vi "feature select.vi"(9 "Feature Selection":T1) -> (3 "VI Refnum":refnum<vi>)   [LabVIEW 2016, in "main.lvlib"]
doc: "Selects which reference is used"
uses:
  main.lvlib
  upper subpanel selection.ctl
  Tools/scan injector.vi
  Tools/Scale - molecular.vi
  Tools/small current measurement.vi
  Tools/GFM monitor.vi
  Features/features/features.lvlib
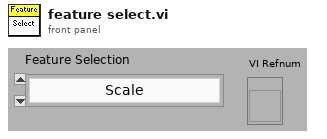
[diagram p1: front panel]
types:
  T1 = typedef "main.lvlib/upper subpanel selection.ctl" = enum16{"Scale", "Injector magnet", "GFM Monitor", "Terminal Voltage", "Source BPM", "Beam Current", "Flat Top", "Scan Injector", "Scale - old"}
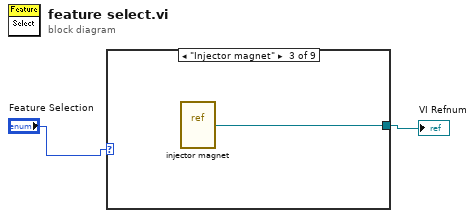
[diagram p0: block diagram]
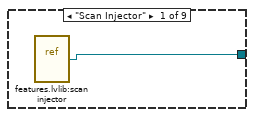
[diagram p2: hidden frame]
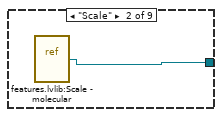
[diagram p3: hidden frame]
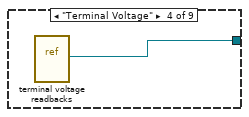
[diagram p4: hidden frame]
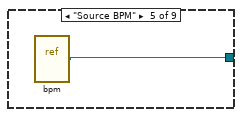
[diagram p5: hidden frame]
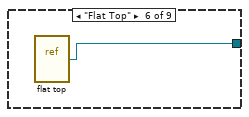
[diagram p6: hidden frame]
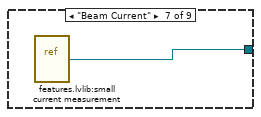
[diagram p7: hidden frame]
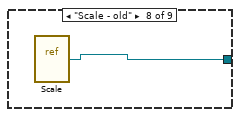
[diagram p8: hidden frame]
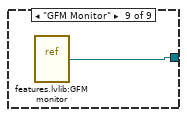
[diagram p9: hidden frame]
diagram:
  n1 = case shown="\"Injector magnet\"" "Feature Selection" {
    tunnel: [w3 w4 w5 w6 w7 w8 w9 w10 w11] -> w1
    frame "Scan Injector" {
      n2 = vi-ref "features.lvlib:scan injector.vi"() -> (w3:refnum<vi>)
    }
    frame "Scale" {
      n3 = vi-ref "features.lvlib:Scale - molecular.vi"() -> (w4:refnum<vi>)
    }
    frame "Injector magnet" {
      n4 = vi-ref "injector magnet.vi"() -> (w5:refnum<vi>)
    }
    frame "Terminal Voltage" {
      n5 = vi-ref "terminal voltage readbacks.vi"() -> (w6:refnum<vi>)
    }
    frame "Source BPM" {
      n6 = vi-ref "bpm.vi"() -> (w7:refnum<vi>)
    }
    frame "Flat Top" {
      n7 = vi-ref "flat top.vi"() -> (w8:refnum<vi>)
    }
    frame "Beam Current" {
      n8 = vi-ref "features.lvlib:small current measurement.vi"() -> (w9:refnum<vi>)
    }
    frame "Scale - old" {
      n9 = vi-ref "Scale.vi"() -> (w10:refnum<vi>)
    }
    frame "GFM Monitor" {
      n10 = vi-ref "features.lvlib:GFM monitor.vi"() -> (w11:refnum<vi>)
    }
  }
  "VI Refnum" <- w1
